vi "Relay Get Refnum (Water Tank).vi"(8 "error in (no error)":errorcluster, 10 "refnum name":string="My Relay RefNum") -> (0 "error out":errorcluster, 3 "RelayDevRef":cluster{string, i32})   [LabVIEW 2013]
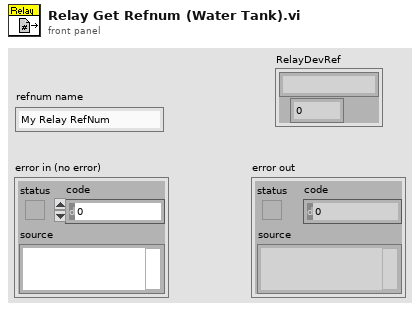
[diagram p1: front panel]
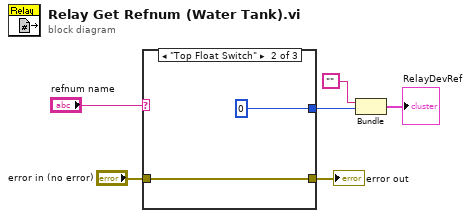
[diagram p0: block diagram]
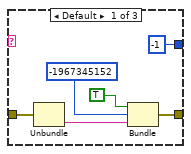
[diagram p2: hidden frame]
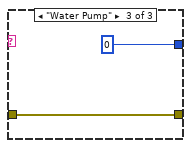
[diagram p3: hidden frame]
diagram:
  n1 = case shown="\"Top Float Switch\"" "refnum name" {
    tunnel: "error in (no error)" -> [w7 w14 w16]
    tunnel: [w8 w14 w16] -> w4
    tunnel: [-1 0 0] -> w2
    frame Default {
      n2 = Unbundle(w7) -> ("source"=w11:string)  [unwired: 2 out]
      n3 = Bundle(TRUE, -1967345152, "source"=w11) -> (w8:cluster{bool, i32, "source":string})  [unwired: 1 in]
    }
    frame "Top Float Switch" {
    }
    frame "Water Pump" {
    }
  }
  "error out" <- w4
  n4 = Bundle("", w2) -> (→"RelayDevRef":cluster{string, i32})  [unwired: 1 in]
